vi "VI Passwortverwaltung.vi"() -> ()   [LabVIEW 2020, in "Passwort.lvlib"]
uses:
  Passwort.lvlib
  Visualisierungs Elemente/Button.ctl
  Passwort Array fuer Anzeige.ctl
  Passwort.ctl
  Visualisierungs Elemente/String - Eingabefeld.ctl
  Visualisierungs Elemente/Zahlen-Eingabefeld.ctl
  FGV Passwort Aktion.ctl
  Allgemein/allgemeine Sub-VIs.lvlib
  Sprachverwaltung/Sprachverwaltung.lvlib
panel:
  in  "Speichern":T1
  in  "Passwortverwaltung":T2 {"Level" format="%#_5g"}
  in  "Stopp":T1
  # "Passwortverwaltung"
  # "Name"
  # "Passwort"
  # "Ebene"
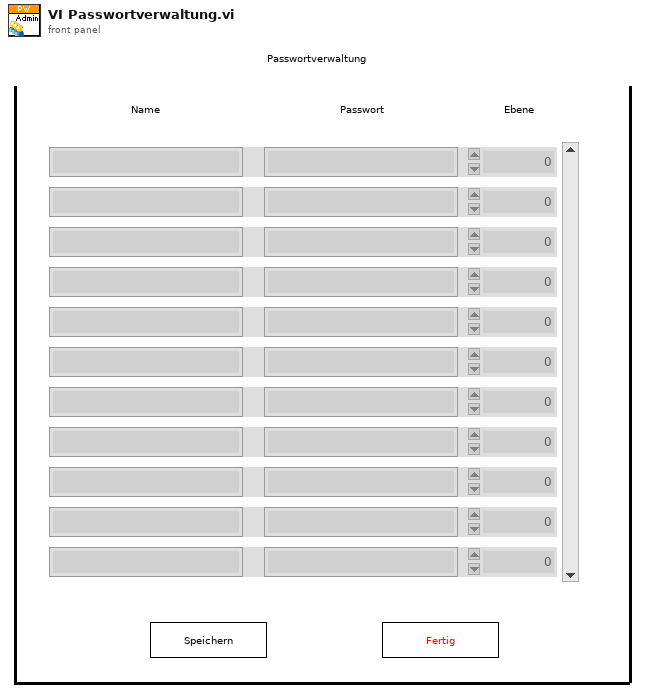
[diagram p1: front panel]
types:
  T1 = typedef "Button.ctl" = bool
  T2 = typedef "Passwort.lvlib/Passwort Array fuer Anzeige.ctl" = T3[]
  T3 = typedef "Passwort.lvlib/Passwort.ctl" = cluster{"Name":T4, "Passwort":T4, "Level":T5}
  T4 = typedef "String - Eingabefeld.ctl" = string
  T5 = typedef "Zahlen-Eingabefeld.ctl" = sgl
  T6 = typedef "Passwort.lvlib/FGV Passwort Aktion.ctl" = enum16{"prüfen", "setzen", "Initialisieren", "PW speichern", "lesen", "PW Änderung"}
  T7 = typedef "Passwort.lvlib/Passwort Array.ctl" = cluster{"Name":string, "Passwort":string, "Level":i16}[]
  T8 = cluster{"Name":string, "Passwort":string, "Level":i16}
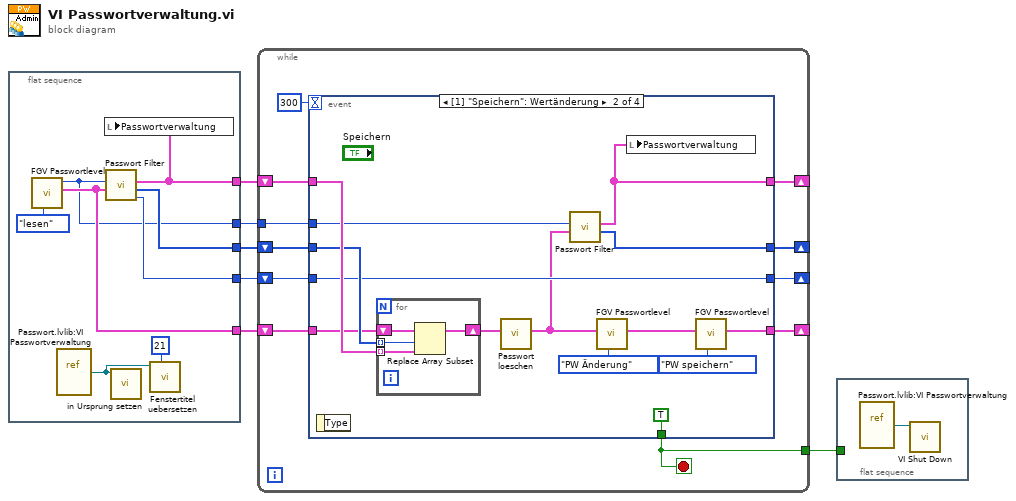
[diagram p0: block diagram]
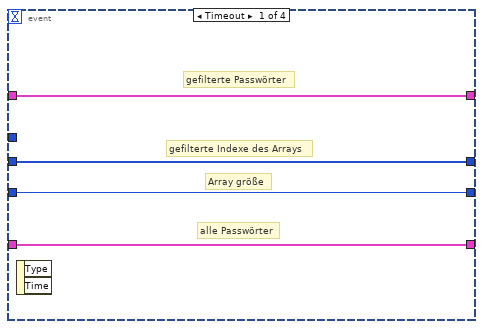
[diagram p2: hidden frame]
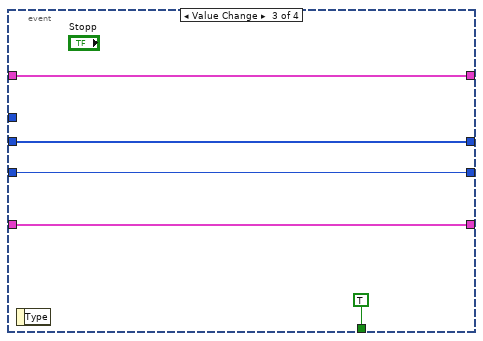
[diagram p3: hidden frame]
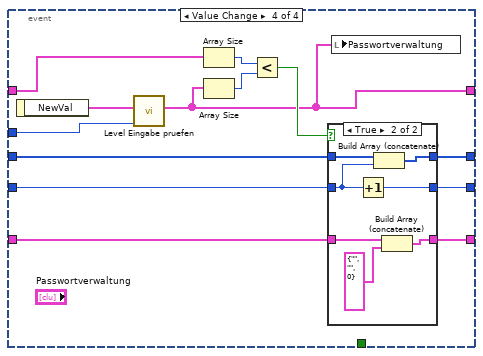
[diagram p4: hidden frame]
diagram:
  n1 = flat-sequence {
    tunnel: [w13] -> w6
    tunnel: [w12] -> w5
    tunnel: [w11] -> w4
    tunnel: [w10] -> w3
    tunnel: [w9] -> w2
    frame #0 {
      n2 = call "FGV Passwortlevel.vi"("FGV Passwort Aktion"=FGV_Passwort_Aktion."lesen") -> ("Passworte"=w11:T7, "aktueller Level"=w9:i16)  [unwired: 8 in, 1 out]
      n3 = vi-ref "Passwort.lvlib:VI Passwortverwaltung.vi"() -> (w8:refnum<vi>)
      n4 = call "Passwort Filter.vi"("Passworte"=w11, "aktueller Level"=w9) -> ("Array Größe"=w10:i32, "gefilterte Indexe"=w12:i32[], "Passworte gefiltert"=w13:T7)  [unwired: 7 in]
      n5 = local write "Passwortverwaltung"(w13) -> ()
      n6 = call "in Ursprung setzen.vi"("VI Referenz"=w8) -> ()  [unwired: 10 in, 1 out]
      n7 = call "Fenstertitel uebersetzen.vi"("Index (Seite)"=21, "Dieses VI"=w8) -> ()  [unwired: 6 in, 4 out]
    }
  }
  n8 = while {
    shift-right: [w24] -> _
    shift-left: w6 -> [w23]
    shift-right: [w20] -> _
    shift-left: w4 -> [w22]
    shift-right: [w17] -> _
    shift-left: w5 -> [w21]
    shift-right: [w18] -> _
    shift-left: w3 -> [w19]
    tunnel: w2 -> [w16]
    tunnel: [w15] -> w1
    stop <- w15 stop-if-true
    n9 = event shown="[1] \"Speichern\": Wertänderung" {
      selector: _ -> [_ _ _ _]
      dyn-events: _ -> [_ _ _ _]
      timeout: 300 -> [_ _ _ _]
      tunnel: [w28 w31 w51 w53] -> w24
      tunnel: w23 -> [w28 w43 w51 w65]
      tunnel: w22 -> [w29 w36 w48 w57]
      tunnel: [w29 w40 w48 w56] -> w20
      tunnel: w21 -> [w27 w42 w50 w61]
      tunnel: [w27 w32 w50 w58] -> w17
      tunnel: w19 -> [w26 w39 w49 w60]
      tunnel: [w26 w39 w49 w59] -> w18
      tunnel: w16 -> [_ w33 _ w54]
      tunnel: [_ TRUE TRUE _] -> w15
      event Timeout {
        # "Array größe"
        # "gefilterte Indexe des Arrays"
        # "alle Passwörter"
        # "gefilterte Passwörter"
        n10 = event-data() -> ()  [unwired: 1 in, 2 out]
      }
      event Value Change {
        n11 = event-data() -> ()  [unwired: 1 in, 1 out]
        n12 = for {
          tunnel: w43 -> [w47] mode=indexing
          tunnel: w42 -> [w46] mode=indexing
          shift-right: [w45] -> w35
          shift-left: w36 -> [w44]
          n13 = Replace Array Subset(array=w44, new element=w47, index=w46) -> (w45:T7)
        }
        n14 = call "Passwort loeschen.vi"("Passworte"=w35) -> ("Passworte"=w34:T7)  [unwired: 10 in]
        n15 = call "Passwort Filter.vi"("Passworte"=w34, "aktueller Level"=w33) -> ("gefilterte Indexe"=w32:i32[], "Passworte gefiltert"=w31:T7)  [unwired: 7 in, 1 out]
        n16 = call "FGV Passwortlevel.vi"("FGV Passwort Aktion"=FGV_Passwort_Aktion."PW Änderung", "Passworte neu"=w34) -> ("Passworte"=w37:T7)  [unwired: 7 in, 2 out]
        n17 = local write "Passwortverwaltung"(w31) -> ()
        n18 = call "FGV Passwortlevel.vi"("FGV Passwort Aktion"=FGV_Passwort_Aktion."PW speichern", "Passworte neu"=w37) -> ("Passworte"=w40:T7)  [unwired: 7 in, 2 out]
      }
      event Value Change {
        n19 = event-data() -> ()  [unwired: 1 in, 1 out]
      }
      event Value Change {
        n20 = event-data() -> ("NewVal"=w55:T2)  [unwired: 1 in]
        n21 = call "Level Eingabe pruefen.vi"("aktueller PW-Level"=w54, "Passworte"=w55) -> ("Passworte"=w53:T7)  [unwired: 9 in]
        n22 = Array Size(array=w65) -> (size(s)=w64:i32)
        n23 = Array Size(array=w53) -> (size(s)=w63:i32)
        n24 = Less?(x=w64, y=w63) -> (x < y?=w62:bool)
        n25 = case shown="True" w62 {
          tunnel: w61 -> [w68 w75]
          tunnel: w60 -> [w67 w74]
          tunnel: [w67 w73] -> w59
          tunnel: [w68 w72] -> w58
          tunnel: w57 -> [w66 w71]
          tunnel: [w66 w69] -> w56
          frame False {
          }
          frame True {
            n26 = Increment(x=w74) -> (x+1=w73:i32)
            n27 = Build Array (concatenate)(w75, w74) -> (w72:i32[])
            n28 = Build Array (concatenate)(w71, T8 {"Name"="", "Passwort"="", "Level"=0} ("Element")) -> (w69:T7)
          }
        }
        n29 = local write "Passwortverwaltung"(w53) -> ()
      }
    }
  }
  n30 = flat-sequence {
    tunnel: w1 -> [_]
    frame #0 {
      n31 = vi-ref "Passwort.lvlib:VI Passwortverwaltung.vi"() -> (w76:refnum<vi>)
      n32 = call "VI Shut Down.vi"("VI Referenz"=w76) -> ()  [unwired: 11 in]
    }
  }
